vi "selecttype.vi"(1 "Conversion Factor Sweep\n1 V = ??":dbl=1.0, 2 "Rate [T/min]":dbl=-1.0 min=-200.0 max=200.0, 3 "DAC number":u8, 4 "Type":string, 5 "To apply":dbl, 6 "error in (no error)":errorcluster, 7 "Fix Instrument":string(combo), 8 "Sweep Instrument":string(combo), 9 "Instrument VISA IN":refnum<visa-resource-name>) -> (0 "error out":errorcluster)   [LabVIEW 2011]
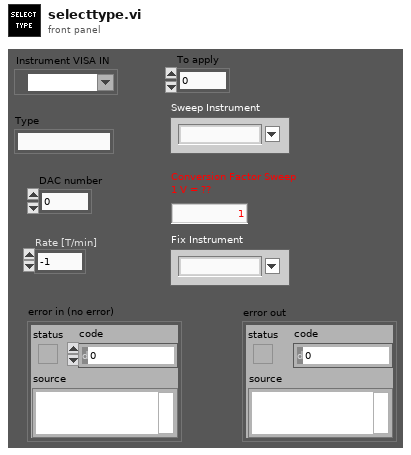
[diagram p1: front panel]
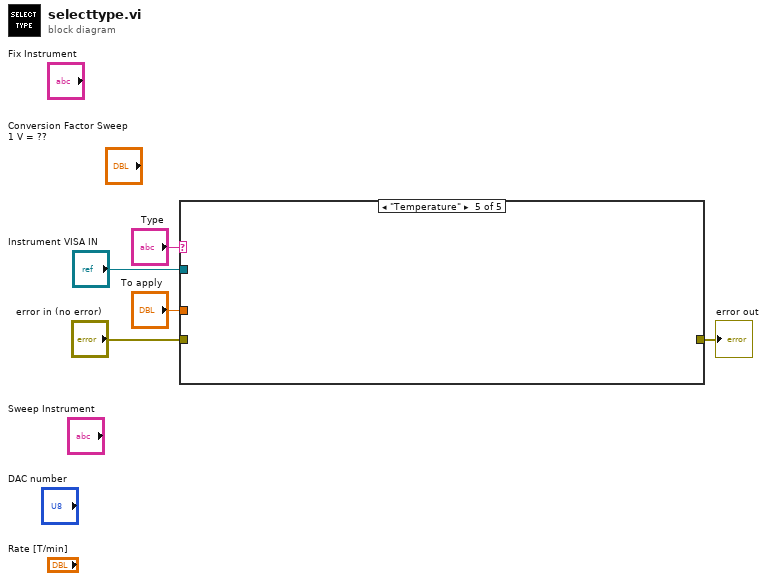
[diagram p0: block diagram]
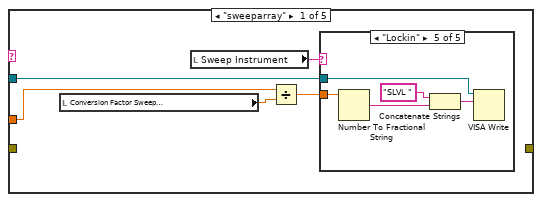
[diagram p2: hidden frame]
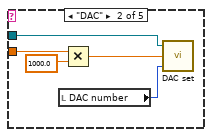
[diagram p4: hidden frame]
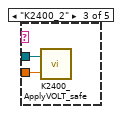
[diagram p5: hidden frame]
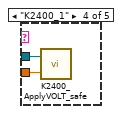
[diagram p6: hidden frame]
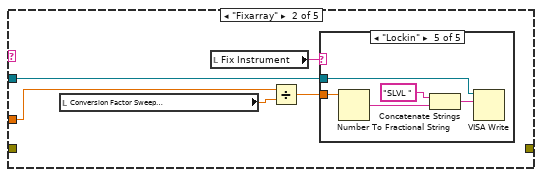
[diagram p7: hidden frame]
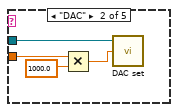
[diagram p9: hidden frame]
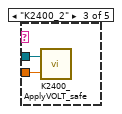
[diagram p10: hidden frame]
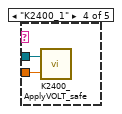
[diagram p11: hidden frame]
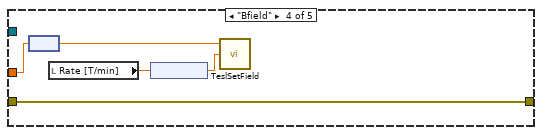
[diagram p13: hidden frame]
diagram:
  n1 = case shown="\"Temperature\"" "Type" {
    tunnel: "Instrument VISA IN" -> [w7 w26 _ _ _]
    tunnel: "error in (no error)" -> [_ _ _ w44 _]
    tunnel: [_ _ _ w44 _] -> w2
    tunnel: "To apply" -> [w6 w25 _ w43 _]
    frame "sweeparray" {
      n2 = local read "Conversion Factor Sweep\n1 V = ??"() -> (w10:dbl)
      n3 = local read "Sweep Instrument"() -> (w8:string)
      n4 = Divide(x=w6, y=w10) -> (x/y=w9:dbl)
      n5 = case shown="\"Lockin\"" w8 {
        tunnel: w9 -> [_ w13 w17 w19 w21]
        tunnel: w7 -> [_ w11 w16 w18 w20]
        frame Default {
        }
        frame "DAC" {
          n6 = local read "DAC number"() -> (w12:u8)
          n7 = Multiply(x=w13, y=1000.0) -> (x*y=w15:dbl)
          n8 = call "DAC set.vi"("DAC number"=w12, "DAC set [mV]"=w15, "DAC COM port"=w11) -> ()  [unwired: 1 out]
        }
        frame "K2400_2" {
          n9 = call "K2400_ApplyVOLT_safe.vi"("Voltage target [V]"=w17, "VISA Resource Name"=w16) -> ()  [unwired: 1 in]
        }
        frame "K2400_1" {
          n10 = call "K2400_ApplyVOLT_safe.vi"("Voltage target [V]"=w19, "VISA Resource Name"=w18) -> ()  [unwired: 1 in]
        }
        frame "Lockin" {
          n11 = Number To Fractional String(number=w21) -> (F-format string=w24:string)  [unwired: 3 out]
          n12 = Concatenate Strings("SLVL " ("chaîne"), w24) -> (w22:string)
          n13 = VISA Write(VISA resource name=w20, write buffer=w22) -> ()  [unwired: 1 in, 3 out]
        }
      }
    }
    frame "Fixarray" {
      n14 = local read "Conversion Factor Sweep\n1 V = ??"() -> (w29:dbl)
      n15 = local read "Fix Instrument"() -> (w27:string)
      n16 = Divide(x=w25, y=w29) -> (x/y=w28:dbl)
      n17 = case shown="\"Lockin\"" w27 {
        tunnel: w28 -> [_ w31 w35 w37 w39]
        tunnel: w26 -> [_ w30 w34 w36 w38]
        frame Default {
        }
        frame "DAC" {
          n18 = Multiply(x=w31, y=1000.0) -> (x*y=w33:dbl)
          n19 = call "DAC set.vi"("DAC set [mV]"=w33, "DAC COM port"=w30) -> ()  [unwired: 1 in, 1 out]
        }
        frame "K2400_2" {
          n20 = call "K2400_ApplyVOLT_safe.vi"("Voltage target [V]"=w35, "VISA Resource Name"=w34) -> ()  [unwired: 1 in]
        }
        frame "K2400_1" {
          n21 = call "K2400_ApplyVOLT_safe.vi"("Voltage target [V]"=w37, "VISA Resource Name"=w36) -> ()  [unwired: 1 in]
        }
        frame "Lockin" {
          n22 = Number To Fractional String(number=w39) -> (F-format string=w42:string)  [unwired: 3 out]
          n23 = Concatenate Strings("SLVL " ("chaîne"), w42) -> (w40:string)
          n24 = VISA Write(VISA resource name=w38, write buffer=w40) -> ()  [unwired: 1 in, 3 out]
        }
      }
    }
    frame Default {
    }
    frame "Bfield" {
      n25 = node(w43) -> (w45:dbl[unit])
      n26 = local read "Rate [T/min]"() -> (w46:dbl)
      n27 = node(w46) -> (w47:dbl[unit])
      n28 = call "TeslSetField.vi"("Sweep rate"=w47, "Field required:"=w45) -> ()  [unwired: 2 in, 2 out]
    }
    frame "Temperature" {
    }
  }
  "error out" <- w2
